vi "7.1-Grab Saitek.vi"() -> (0 "Saitek ID":refnum<k1>)   [LabVIEW 2011]
uses:
  <vilib>/regexp/Match Regular Expression.xnode
panel:
  out "whole match":string
  out "device name":string
  out "joystick info":T1(array[cluster])
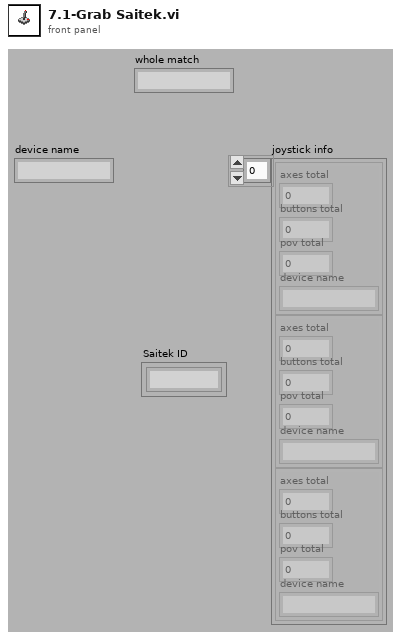
[diagram p1: front panel]
types:
  T1 = cluster{"axes total":u32, "buttons total":u32, "pov total":u32, "device name":string}[]
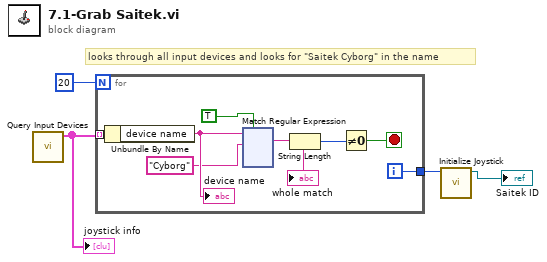
[diagram p0: block diagram]
diagram:
  # "looks through all input devices and looks for \"Saitek Cyborg\" in the name"
  n1 = call <vilib>:"Query Input Devices.vi"() -> ("joystick info"=w1:T1)  [unwired: 8 in, 3 out]
  "joystick info" <- w1
  n2 = for {
    N: 20 -> [_]
    tunnel: w1 -> [w12] mode=indexing
    tunnel: [w5] -> w4
    i -> [w5]
    stop <- w6 stop-if-true
    n3 = Unbundle By Name(w12) -> ("device name"=w11:string)
    "device name" <- w11
    n4 = xnode "Match Regular Expression"("input string"=w11, "regular expression"="Cyborg", "ignore case? (F)"=TRUE) -> ("whole match"=w8:string)  [unwired: 3 in, 4 out]
    "whole match" <- w8
    n5 = String Length(string=w8) -> (length=w7:i32)
    n6 = Not Equal To 0?(x=w7) -> (x != 0?=w6:bool)
  }
  n7 = call <vilib>:"Initialize Joystick.vi"("device index"=w4) -> ("device ID"=→"Saitek ID":refnum<k1>)  [unwired: 9 in, 1 out]
